vi "Publisher.vi"() -> ()   [LabVIEW 2014]
uses:
  <vilib>/ptbypt/NI_PtbyPt.lvlib
  lvnanomsg/nanomsg_context.lvclass
  lvnanomsg/nanomsg_socket.lvclass
panel:
  out "Numeric":u64
  out "dT":u32
  out "Waveform Chart":dbl(graph)
  in  "milliseconds to wait":u32=100
  in  "stop 2":bool
  in  "endpoint":string="tcp://192.168.3.98:55555"
  out "error IO":errorcluster
  in  "stop":bool
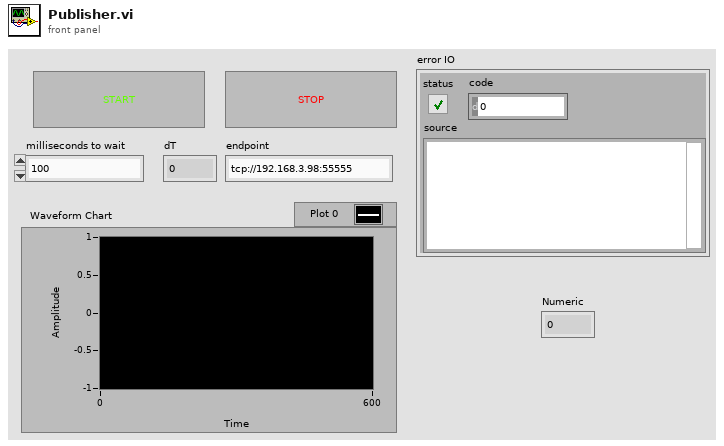
[diagram p1: front panel]
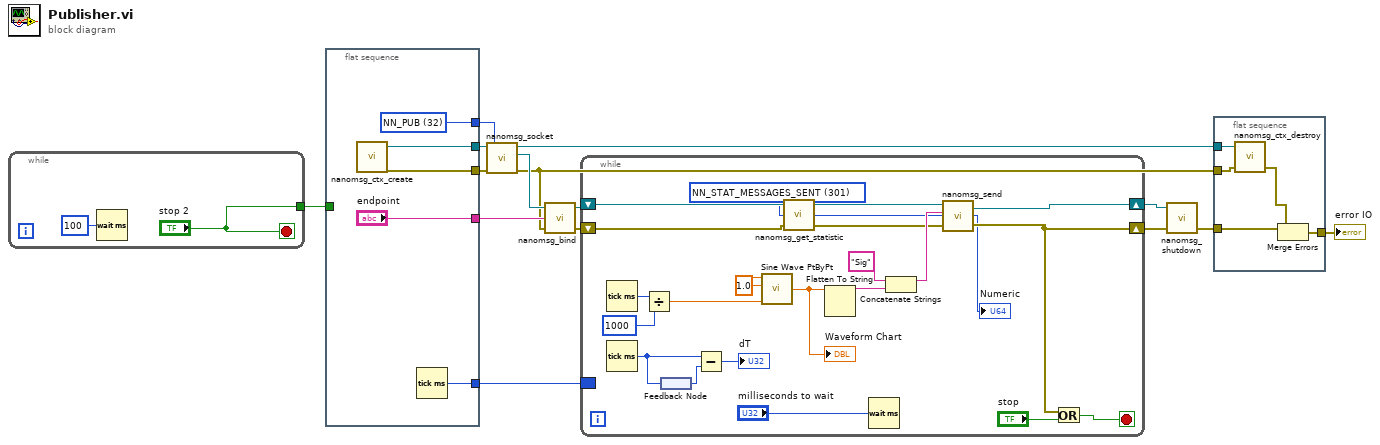
[diagram p0: block diagram]
diagram:
  n1 = while {
    tunnel: ["stop 2"] -> w3
    stop <- "stop 2" stop-if-true
    n2 = Wait (ms)(milliseconds to wait=u32 100) -> ()  [unwired: 1 out]
  }
  n3 = flat-sequence {
    tunnel: [w22] -> w14
    tunnel: [w21] -> w6
    tunnel: [w20] -> w5
    tunnel: ["endpoint"] -> w4
    tunnel: w3 -> [_]
    tunnel: [w18] -> w2
    frame #0 {
      w22 = 32 items=["NN_WS"=-4, "NN_TCP"=-3, "NN_IPC"=-2, "NN_INPROC"=-1, "NN_SOL_SOCKET"=0, "NN_PAIR"=16, "NN_PUB"=32, "NN_SUB"=33, "NN_REQ"=48, "NN_REP"=49, "NN_PUSH"=80, "NN_PULL"=81, "NN_SURVEYOR"=98, "NN_RESPONDENT"=99, "NN_BUS"=112] ("socket type")
      n4 = call "nanomsg_ctx_create.vi"() -> ("error out"=w20:errorcluster, "context out"=w21:refnum<class "nanomsg_context.lvclass">)  [unwired: 4 in]
      n5 = Tick Count (ms)() -> (millisecond timer value=w18:u32)
    }
  }
  n6 = call "nanomsg_socket.vi"("error in"=w5, "socket type"=w14, "context in"=w6) -> ("error out"=w1:errorcluster, "socket out"=w13:refnum<class "nanomsg_socket.lvclass">, "context out"=w15:refnum<class "nanomsg_context.lvclass">)  [unwired: 2 in]
  n7 = call "nanomsg_bind.vi"("error in"=w1, "endpoint"=w4, "socket in"=w13) -> ("error out"=w11:errorcluster, "socket out"=w12:refnum<class "nanomsg_socket.lvclass">)  [unwired: 1 in]
  n8 = while {
    shift-right: [w39] -> w10
    shift-left: w12 -> [w41]
    shift-right: [w40] -> w9
    shift-left: w11 -> [w26]
    border: w2 -> [_]
    stop <- w42 stop-if-true
    w24 = 301 items=["NN_STAT_ESTABLISHED_CONNECTIONS"=101, "NN_STAT_ACCEPTED_CONNECTIONS"=102, "NN_STAT_DROPPED_CONNECTIONS"=103, "NN_STAT_BROKEN_CONNECTIONS"=104, "NN_STAT_CONNECT_ERRORS"=105, "NN_STAT_BIND_ERRORS"=106, "NN_STAT_ACCEPT_ERRORS"=107, "NN_STAT_CURRENT_CONNECTIONS"=201, "NN_STAT_INPROGRESS_CONNECTIONS"=202, "NN_STAT_CURRENT_EP_ERRORS"=203, "NN_STAT_MESSAGES_SENT"=301, "NN_STAT_MESSAGES_RECEIVED"=302, "NN_STAT_BYTES_SENT"=303, "NN_STAT_BYTES_RECEIVED"=304, "NN_STAT_CURRENT_SND_PRIORITY"=401] ("statistics type")
    w31 = 1.0 ("frequency")
    n9 = Tick Count (ms)() -> (millisecond timer value=w35:u32)
    n10 = Tick Count (ms)() -> (millisecond timer value=w30:u32)
    n11 = Divide(x=w35, y=u32 1000) -> (x/y=w32:dbl)
    n12 = feedback #1() -> (w29:u32)
    n13 = feedback-in #1(w30) -> ()
    n14 = Subtract(x=w30, y=w29) -> (x-y=→"dT":u32)
    n15 = call <vilib>:"Sine Wave PtByPt.vi"("time"=w32, "frequency"=w31, "amplitude"=w31) -> ("sine wave"=w33:dbl)  [unwired: 1 in]
    "Waveform Chart" <- w33
    n16 = call "nanomsg_get_statistic.vi"("error in"=w26, "statistic"=w24, "socket in"=w41) -> ("error out"=w25:errorcluster, "result"=→"Numeric":u64, "socket out"=w27:refnum<class "nanomsg_socket.lvclass">)
    n17 = Flatten To String(anything=w33) -> (data string=w36:string)  [unwired: 3 in, 2 out]
    n18 = Wait (ms)(milliseconds to wait="milliseconds to wait") -> ()  [unwired: 1 out]
    n19 = Concatenate Strings("Sig" ("string"), w36) -> (w37:string)
    n20 = call "nanomsg_send.vi"("error in"=w25, "data"=w37, "socket in"=w27) -> ("error out"=w40:errorcluster, "socket out"=w39:refnum<class "nanomsg_socket.lvclass">)  [unwired: 1 in]
    n21 = Or(x=w40, y="stop") -> (x .or. y?=w42:bool)
  }
  n22 = call "nanomsg_shutdown.vi"("error in"=w9, "socket"=w10) -> ("error out"=w8:errorcluster)  [unwired: 3 in]
  n23 = flat-sequence {
    tunnel: w15 -> [w46]
    tunnel: w8 -> [w49]
    tunnel: [w47] -> w7
    tunnel: w1 -> [w45]
    frame #0 {
      n24 = call "nanomsg_ctx_destroy.vi"("error in"=w45, "context in"=w46) -> ("error out"=w48:errorcluster)  [unwired: 3 in]
      n25 = Merge Errors(w49, w48) -> (w47:errorcluster)
    }
  }
  "error IO" <- w7
